vi "_PC_SaveFile setXYGraphAttr.vi"(8 "error in (no error)":errorcluster, 9 "plot name":string[](array[string]), 10 "plot value":cluster{"X":dbl[], "Y":sgl[]}[](array[cluster]), 11 "graph in":refnum<vi>) -> (0 "error out":errorcluster, 3 "graph out":refnum<vi>)   [LabVIEW 2018]
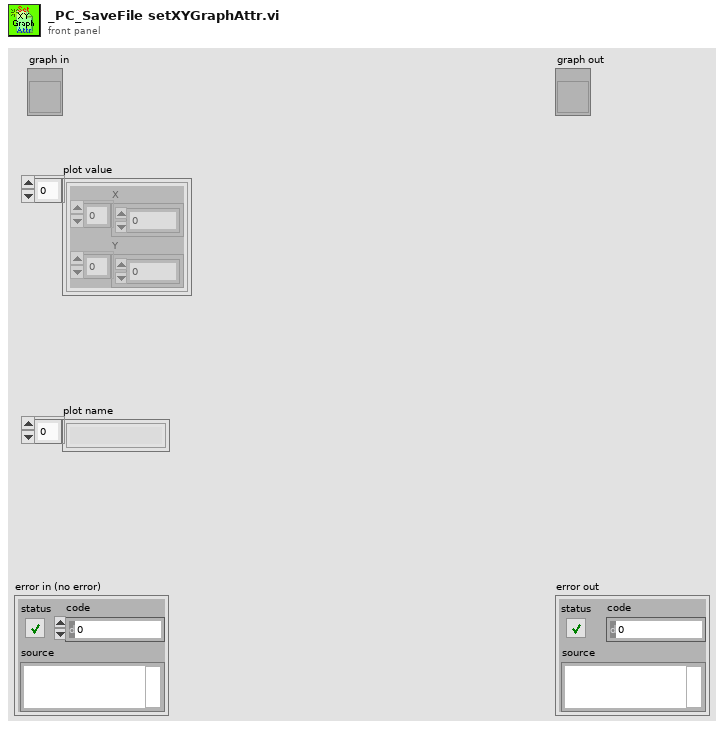
[diagram p1: front panel]
types:
  T1 = cluster{"BGColor":u32, "GridX":bool, "GridY":bool, "LineColorArray":u32[], "LineWidthArray":u8[]}
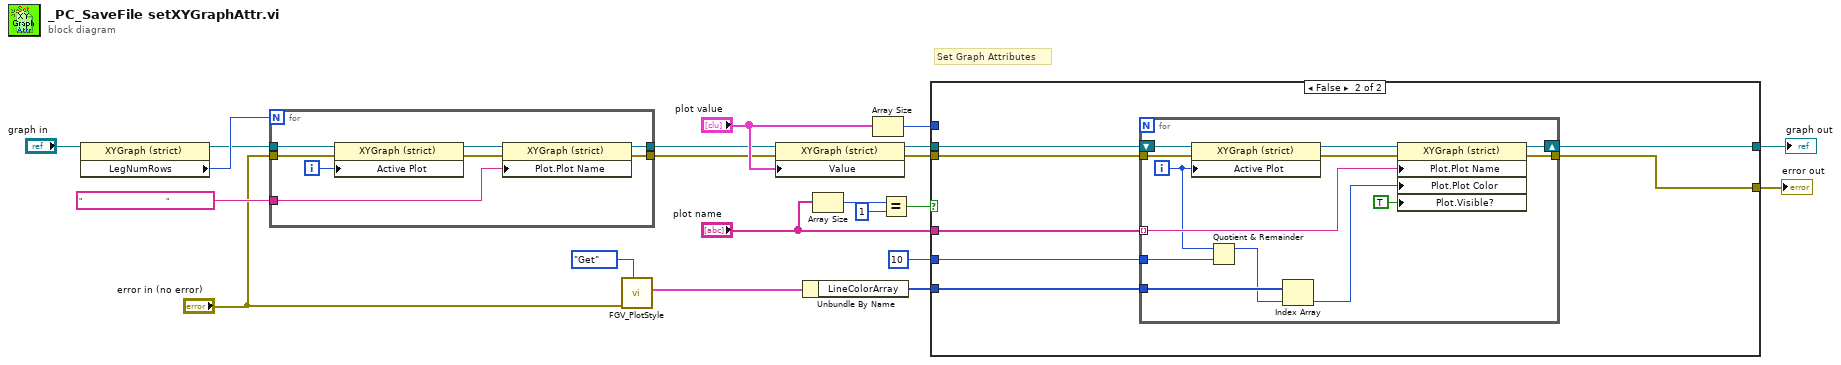
[diagram p0: block diagram]
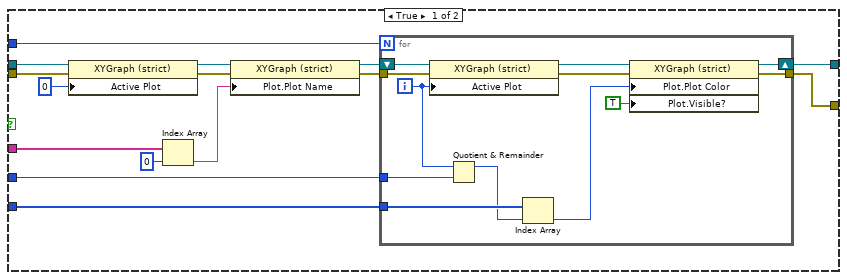
[diagram p2: hidden frame]
diagram:
  # "Set Graph Attributes"
  n1 = property class="XYGraph (strict)"(reference="graph in") -> (reference out=w1:refnum<vi>, "LegNumRows"=w2:u32)  [unwired: 1 in, 1 out]
  n2 = for {
    N: w2 -> [_]
    tunnel: w1 -> [w29]
    tunnel: "                                          " -> [w27]
    tunnel: [w24] -> w7
    tunnel: "error in (no error)" -> [w23]
    tunnel: [w22] -> w8
    i -> [w28]
    n3 = property class="XYGraph (strict)"(reference=w29, error in=w23, "Active Plot"=w28) -> (reference out=w26:refnum<vi>, error out=w25:errorcluster)
    n4 = property class="XYGraph (strict)"(reference=w26, error in=w25, "Plot.Plot Name"=w27) -> (reference out=w24:refnum<vi>, error out=w22:errorcluster)
  }
  n5 = call "FGV_PlotStyle.vi"("Function"=enum16{"Set", "Get"}."Get", "error in (no error)"="error in (no error)") -> ("Output Cluster"=w20:T1)  [unwired: 8 in, 1 out]
  n6 = property class="XYGraph (strict)"(reference=w7, error in=w8, "Value"="plot value") -> (reference out=w15:refnum<vi>, error out=w14:errorcluster)
  n7 = Unbundle By Name(w20) -> ("LineColorArray"=w19:u32[])
  n8 = Array Size(array="plot name") -> (size(s)=w18:i32)
  n9 = Array Size(array="plot value") -> (size(s)=w12:i32)
  n10 = Equal?(x=w18, y=1) -> (x = y?=w16:bool)
  n11 = case shown="False" w16 {
    tunnel: w15 -> [w41 w63]
    tunnel: 10 -> [w44 w62]
    tunnel: w19 -> [w43 w61]
    tunnel: [w42 w60] -> w6
    tunnel: "plot name" -> [w37 w59]
    tunnel: w14 -> [w32 w58]
    tunnel: w12 -> [w31 _]
    tunnel: [w30 w57] -> w4
    frame True {
      n12 = property class="XYGraph (strict)"(reference=w41, error in=w32, "Active Plot"=u32 0) -> (reference out=w39:refnum<vi>, error out=w38:errorcluster)
      n13 = Index Array(array=w37, index=0) -> (element=w35:string)
      n14 = property class="XYGraph (strict)"(reference=w39, error in=w38, "Plot.Plot Name"=w35) -> (reference out=w34:refnum<vi>, error out=w33:errorcluster)
      n15 = for {
        N: w31 -> [_]
        tunnel: [w54] -> w42
        tunnel: w43 -> [w50]
        tunnel: w44 -> [w51]
        tunnel: w33 -> [w49]
        shift-right: [w45] -> w30
        shift-left: w34 -> [w56]
        i -> [w52]
        n16 = property class="XYGraph (strict)"(reference=w56, error in=w49, "Active Plot"=w52) -> (reference out=w55:refnum<vi>, error out=w53:errorcluster)
        n17 = Quotient & Remainder(x=w52, y=w51) -> (x-y*floor(x/y)=w48:i32)  [unwired: 1 out]
        n18 = Index Array(array=w50, index=w48) -> (element=w47:u32)
        n19 = property class="XYGraph (strict)"(reference=w55, error in=w53, "Plot.Plot Color"=w47, "Plot.Visible?"=TRUE ("Plot.Visible")) -> (reference out=w45:refnum<vi>, error out=w54:errorcluster)
      }
    }
    frame False {
      n20 = for {
        tunnel: w59 -> [w74] mode=indexing
        tunnel: [w73] -> w60
        tunnel: w61 -> [w69]
        tunnel: w62 -> [w70]
        tunnel: w58 -> [w66]
        shift-right: [w64] -> w57
        shift-left: w63 -> [w76]
        i -> [w71]
        n21 = property class="XYGraph (strict)"(reference=w76, error in=w66, "Active Plot"=w71) -> (reference out=w75:refnum<vi>, error out=w72:errorcluster)
        n22 = Quotient & Remainder(x=w71, y=w70) -> (x-y*floor(x/y)=w67:i32)  [unwired: 1 out]
        n23 = Index Array(array=w69, index=w67) -> (element=w68:u32)
        n24 = property class="XYGraph (strict)"(reference=w75, error in=w72, "Plot.Plot Name"=w74, "Plot.Plot Color"=w68, "Plot.Visible?"=TRUE ("Plot.Visible")) -> (reference out=w64:refnum<vi>, error out=w73:errorcluster)
      }
    }
  }
  "error out" <- w6
  "graph out" <- w4
